vi "True at one time of day.vi"(9 "Next start time in":dbl, 10 "Time stamp from INI (only will use time Not date)":timestamp=timestamp(3379345619.5334554 s since 1904-01-01)) -> (0 "error out":errorcluster, 1 "next start time out":dbl caption="Get Start Time (s)", 2 "Time Until Next Scan (H)":dbl caption="Elapsed Time (s)" format="%#_2g", 3 "Time has Elapsed":bool=TRUE)   [LabVIEW 2011]
uses:
  <vilib>/Utility/miscctls.llb/LVDateTimeRec.ctl
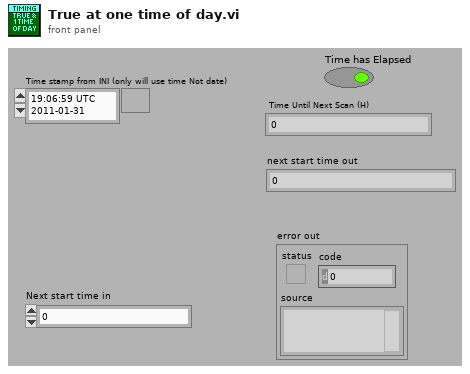
[diagram p1: front panel]
types:
  T1 = typedef "LVDateTimeRec.ctl" = cluster{"fractional second":dbl, "second":i32, "minute":i32, "hour":i32, "day of month":i32, "month":i32, "year":i32, "day of week":i32, "day of year":i32, "DST":i32}
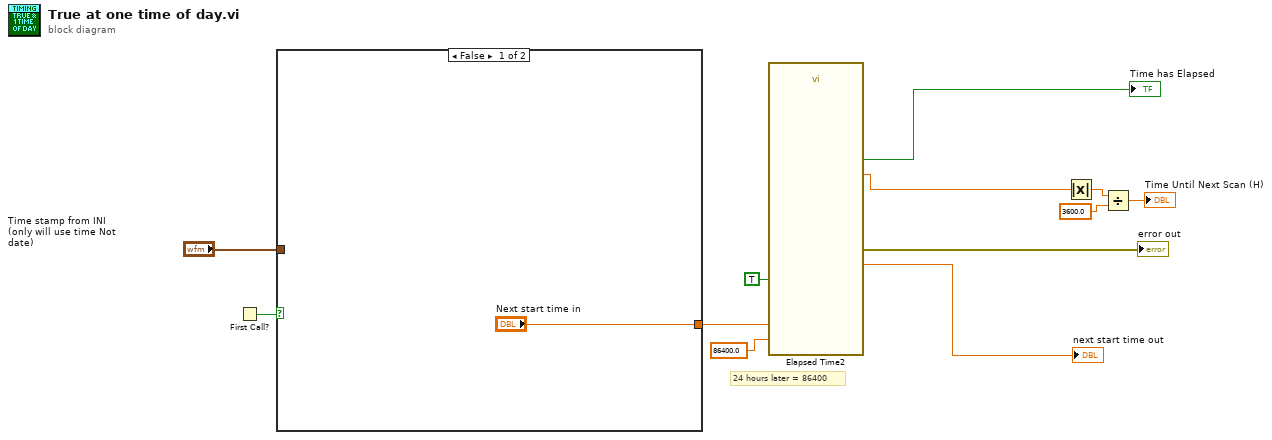
[diagram p0: block diagram]
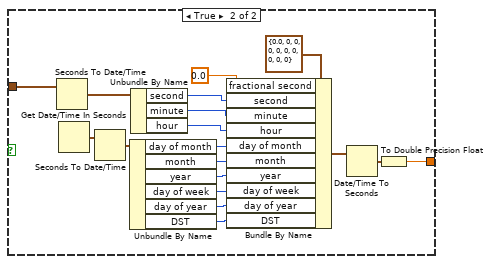
[diagram p2: hidden frame]
diagram:
  # "24 hours later = 86400"
  n1 = First Call?() -> (First Call?: T/F=w4:bool)
  n2 = case shown="False" w4 {
    tunnel: ["Next start time in" w30] -> w6
    tunnel: "Time stamp from INI (only will use time Not date)" -> [_ w29]
    frame False {
    }
    frame True {
      n3 = Seconds To Date/Time(time stamp (now)=w29) -> (date time rec=w22:T1)  [unwired: 1 in]
      n4 = Get Date/Time In Seconds() -> (seconds since 1Jan1904=w15:timestamp)
      n5 = Seconds To Date/Time(time stamp (now)=w15) -> (date time rec=w14:T1)  [unwired: 1 in]
      n6 = Unbundle By Name(w14) -> ("day of month"=w16:i32, "month"=w27:i32, "year"=w26:i32, "day of week"=w25:i32, "day of year"=w24:i32, "DST"=w23:i32)
      n7 = Unbundle By Name(w22) -> ("second"=w21:i32, "minute"=w20:i32, "hour"=w19:i32)
      n8 = Bundle By Name(cluster=T1 {"fractional second"=0.0, "second"=0, "minute"=0, "hour"=0, "day of month"=0, "month"=0, "year"=0, "day of week"=0, "day of year"=0, "DST"=0} ("date time rec 2"), "fractional second"=0.0, "second"=w21, "minute"=w20, "hour"=w19, "day of month"=w16, "month"=w27, "year"=w26, "day of week"=w25, "day of year"=w24, "DST"=w23) -> (w17:T1)
      n9 = Date/Time To Seconds(2:w17) -> (0:w31:timestamp)  [unwired: 1 in]
      n10 = To Double Precision Float(number=w31) -> (double precision float=w30:dbl)
    }
  }
  n11 = call "Elapsed Time2"("Time Target (s)"=86400.0, "Auto Reset"=TRUE, "Set Start Time (s)"=w6) -> ("Get Start Time (s)"=→"next start time out":dbl, "Elapsed Time (s)"=w8:dbl, "Time has Elapsed"=→"Time has Elapsed":bool, "error out"=→"error out":errorcluster)  [unwired: 9 in, 4 out]
  n12 = Absolute Value(x=w8) -> (abs(x)=w7:dbl)
  n13 = Divide(x=w7, y=3600.0) -> (x/y=→"Time Until Next Scan (H)":dbl)
